vi "Module - LINX.vi"(8 "error in (no error)":errorcluster) -> (0 "error out":errorcluster)   [LabVIEW 2020]
uses:
  Control/State - LINX.ctl
  <vilib>/MakerHub/LINX/Private/Type Defs/LINX Ref.ctl
  <vilib>/MakerHub/LINX/Private/Type Defs/Platform.ctl
  <vilib>/MakerHub/LINX/Private/Type Defs/Interface.ctl
  <vilib>/MakerHub/LINX/Private/Device/Type Defs/LINX Device Config.ctl
  <vilib>/MakerHub/LINX/Private/Device/Type Defs/TCP Config.ctl
  <vilib>/MakerHub/LINX/Private/Device/Type Defs/Channels.ctl
  <vilib>/MakerHub/LINX/Private/Device/Type Defs/Wifi Config.ctl
  <vilib>/MakerHub/LINX/Private/Type Defs/WIFI Security Type.ctl
  Control/MQTT Received Data.ctl
  Control/Config File Section List.ctl
  Shared/Control/State - eFGV.ctl
  Control/MQTT Send Data.ctl
  <vilib>/numeric/Random Number (Range) U64.vi
  a823c940-d7b3-4362-9922-b3ec767b4119.vi
  <vilib>/MakerHub/LINX/Public/Peripherals/Digital/Digital Read N Chans.vi
  <vilib>/numeric/sub_Random U32.vi
  <vilib>/MakerHub/LINX/Private/Local IO/LinxDigitalRead.vi
  <vilib>/MakerHub/LINX/Public/Utilities/Check Channel.vi
  <vilib>/MakerHub/LINX/Private/Local IO/Handle Errors.vi
  <vilib>/MakerHub/LINX/Public/Utilities/Open Local.vi
  <vilib>/MakerHub/LINX/Private/Utilties/Generate Error.vi
  <userlib>/_OpenG.lib/comparison/comparison.llb/I32 Changed__ogtk.vi
  <vilib>/Comparison/Equal/Equal Functor/Equal Functor.lvclass
  <vilib>/MakerHub/LINX/LMH-LINX.lvlib
  <vilib>/MakerHub/LINX/Private/Device/Device.lvlib
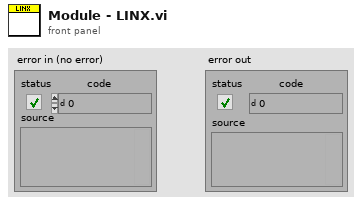
[diagram p1: front panel]
types:
  T1 = typedef "LMH-LINX.lvlib/LINX Ref.ctl" = cluster{"IO":T2, "Interface":T3, "LINX Device Config":T4}
  T2 = typedef "LMH-LINX.lvlib/Platform.ctl" = enum16{"Remote", "Local"}
  T3 = typedef "LMH-LINX.lvlib/Interface.ctl" = enum16{"Serial", "TCP"}
  T4 = typedef "LMH-LINX.lvlib/Device.lvlib/LINX Device Config.ctl" = cluster{"Interface":T3, "COM Port":refnum<visa-resource-name>, "TCP Configuration":T5, "Device Family":u8, "Device ID":u8, "Device Name":string, "TCP Ref":refnum<k5>, "Channels":T6}
  T5 = typedef "LMH-LINX.lvlib/Device.lvlib/TCP Config.ctl" = cluster{"IP Address":string, "Port":u16}
  T6 = typedef "LMH-LINX.lvlib/Channels.ctl" = cluster{"DI":u8[], "DO":u8[], "AI":u8[], "AO":u8[], "PWM":u8[], "QE":u8[], "UART":u8[], "I2C 2":u8[], "SPI":u8[], "CAN":u8[], "Servo":u8[], "AI Ref (V)":dbl, "AI Resolution (Bits)":u8, "AO Ref (V)":dbl, "AO Resolution (Bits)":u8}
  T7 = typedef "LMH-LINX.lvlib/Device.lvlib/Wifi Config.ctl" = cluster{"SSID":string, "IP Address":string, "Port":u16, "WIFI Security Type":T8, "Password":string}
  T8 = typedef "LMH-LINX.lvlib/WIFI Security Type.ctl" = enum8{"None", "WPA2 Password", "WPA2 Key", "WEP40", "WEP104"}
  T9 = typedef "MQTT Received Data.ctl" = cluster{"Receiving Module":string, "Topic":string, "Data":variant}
  T10 = cluster{"TOut":i32, "Module Name":string, "LINX Connected":bool, "User exit":bool, "Device Name":string, "LINX Resource":T1, "Wifi Configuration":T7, "Pass Counter":i32, "Reject Counter":i32, "MQTT Received Data":T9, "CK ID List":string[], "CK Defect List":string[], "CK Reject List":string[], "ID Present":bool, "Pulse per rotation":i32, "CK ID":string, "Is CK Pass?":bool, "CK ID Index":i32, "Is CK Interlock?":bool, "Extension":string}
  T11 = typedef "State - LINX.ctl" = enum16{"Init module", "Read config file", "Register for event", "Idle", "Transmit ID to Server", "Check ID in List", "Handle MQTT Event", "Create LINX Ref", "Read LINX - Digital In", "Write CK Pass", "Destroy LINX Ref", "Unregister user event", "Close module"}
  T12 = typedef "Config File Section List.ctl" = enum16{"RasPi Setting", "MQTT Server Setting", "MQTT Client Setting", "WiFi Setting", "MQTT Topics"}
  T13 = typedef "State - eFGV.ctl" = enum16{"Init", "Read", "Write", "Close"}
  T14 = typedef "MQTT Send Data.ctl" = cluster{"Sender Module":string, "Receiving Module":string, "Topic":string, "Data":variant}
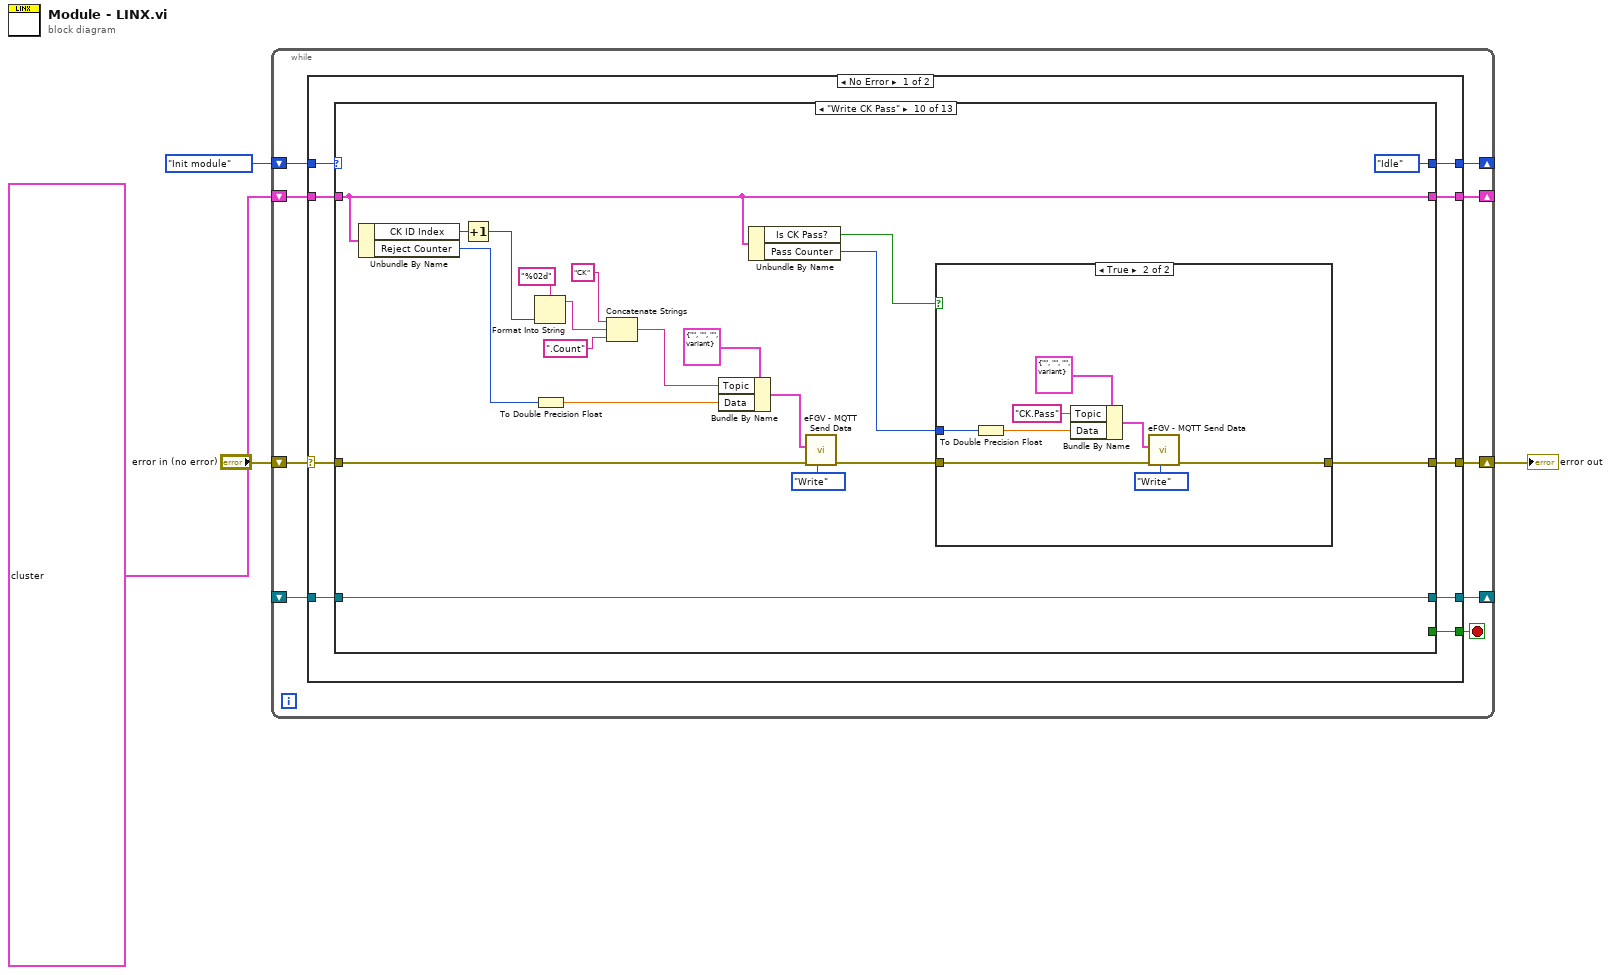
[diagram p0: block diagram]
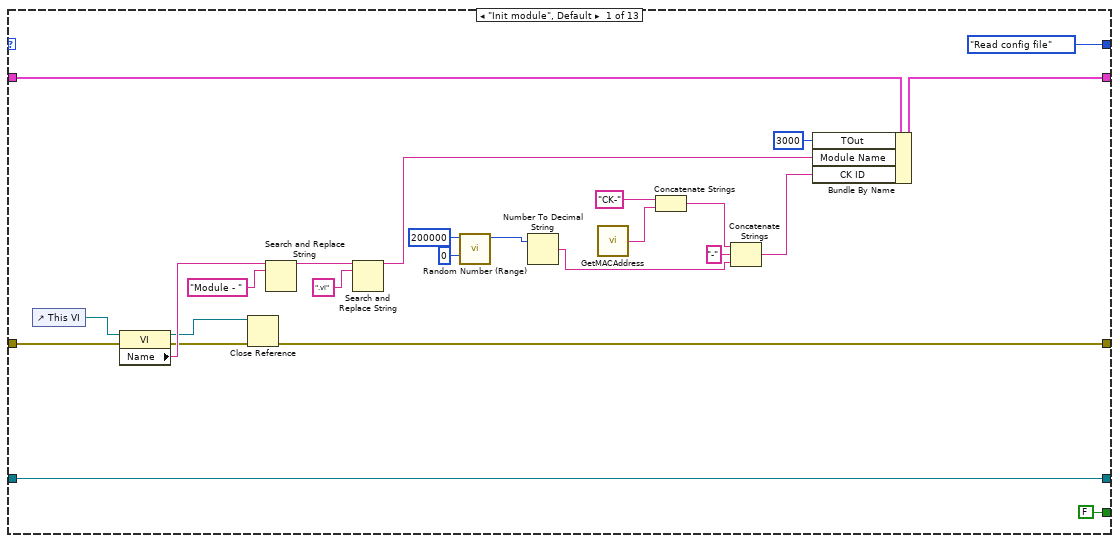
[diagram p2: hidden frame]
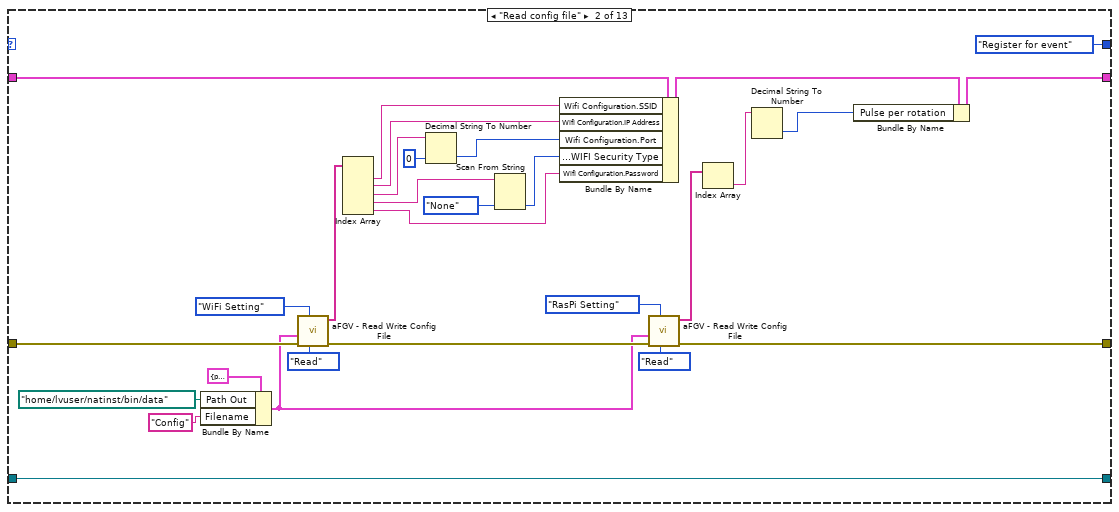
[diagram p3: hidden frame]
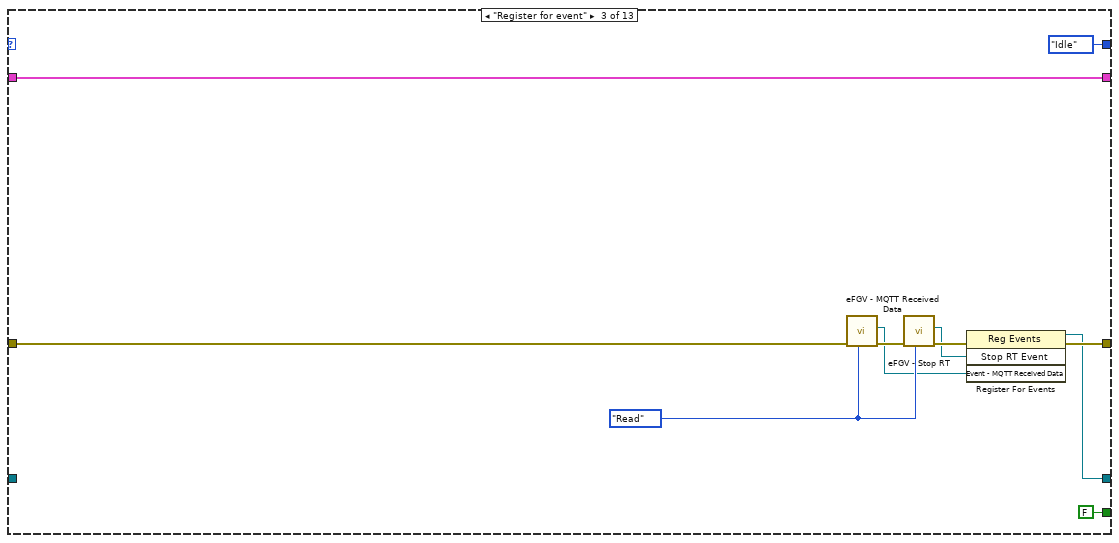
[diagram p4: hidden frame]
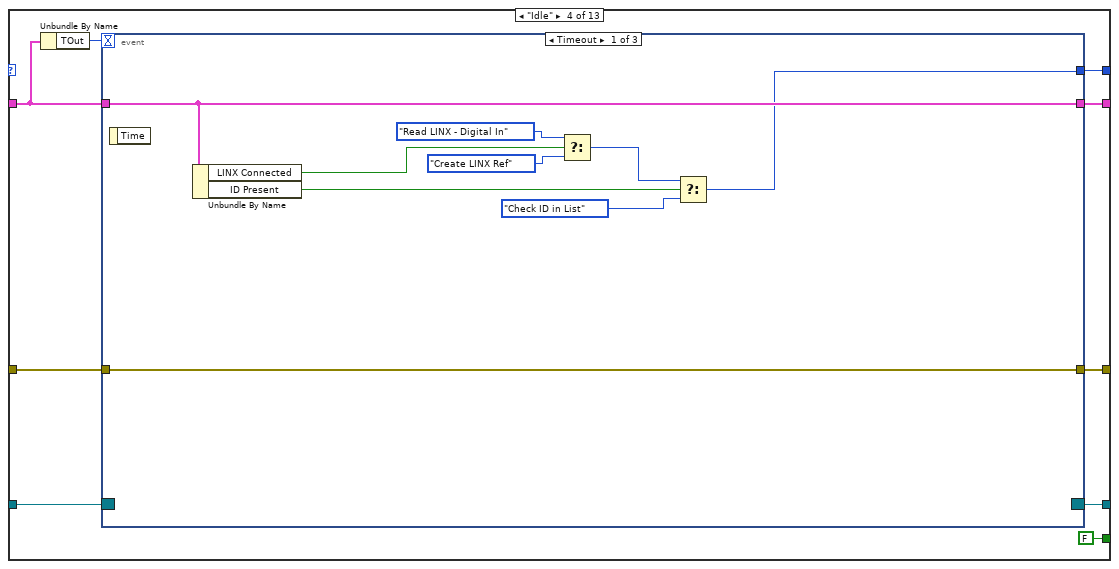
[diagram p5: hidden frame]
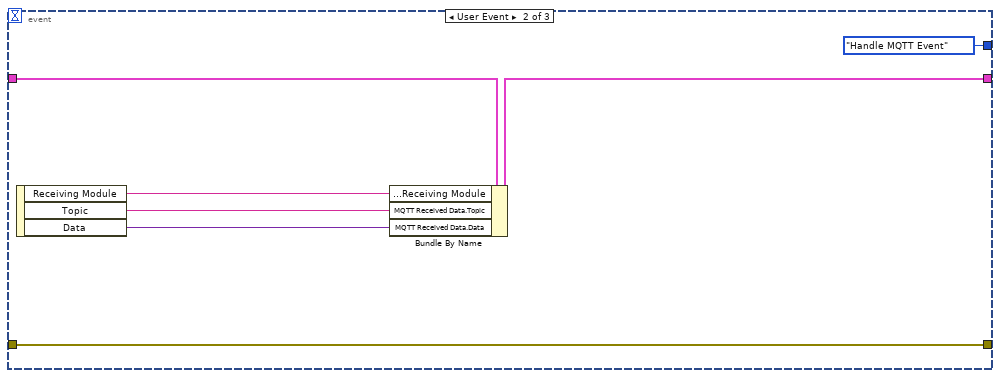
[diagram p6: hidden frame]
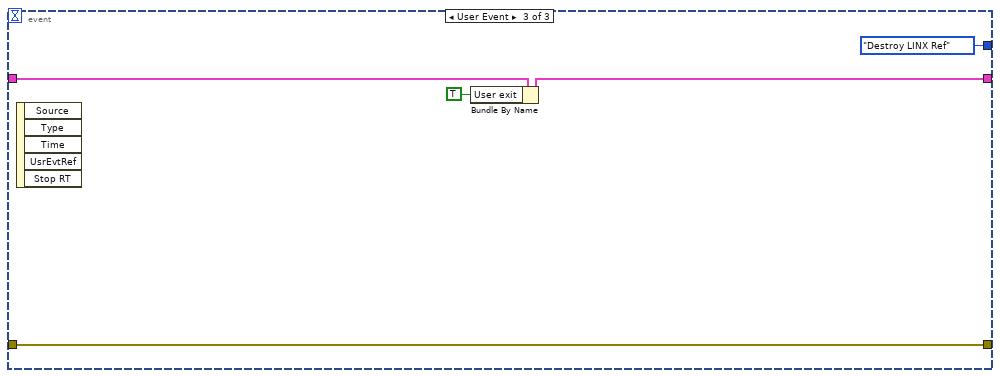
[diagram p7: hidden frame]
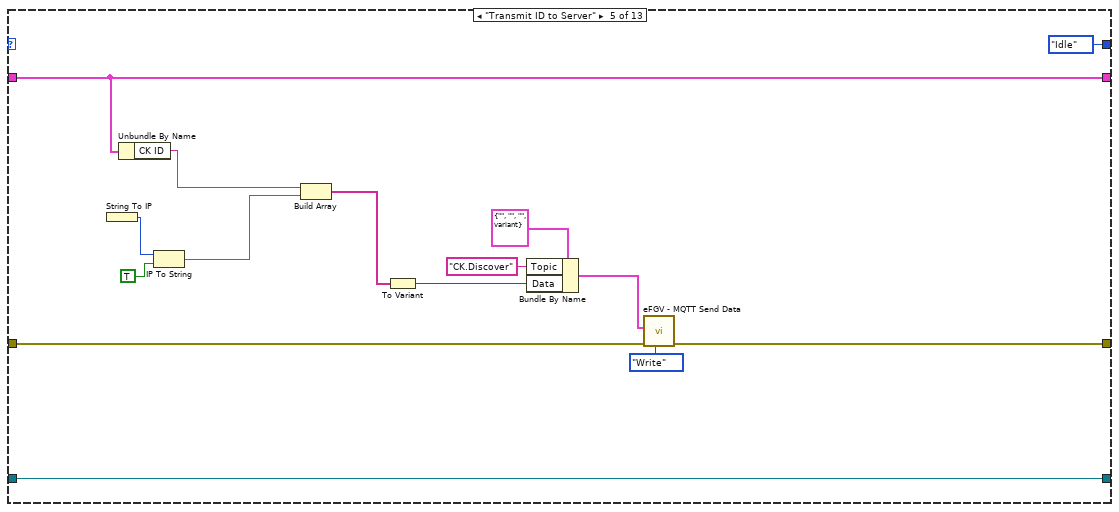
[diagram p8: hidden frame]
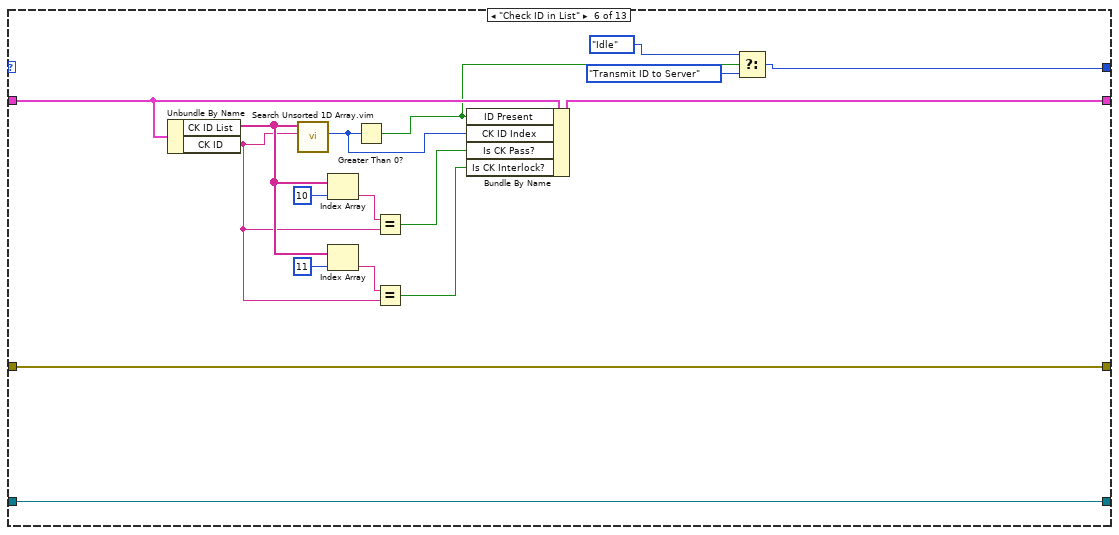
[diagram p9: hidden frame]
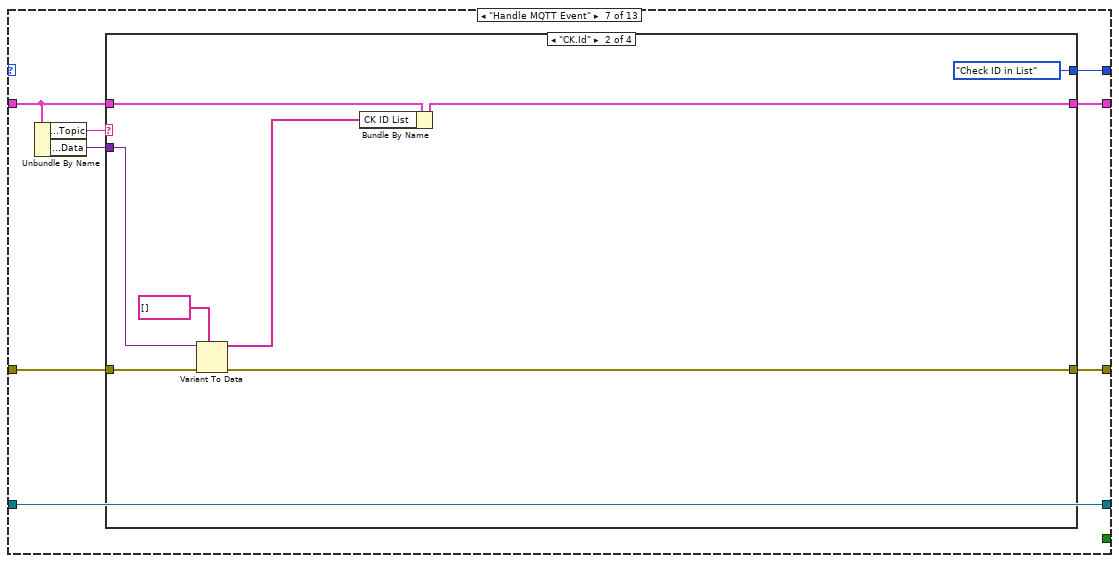
[diagram p10: hidden frame]
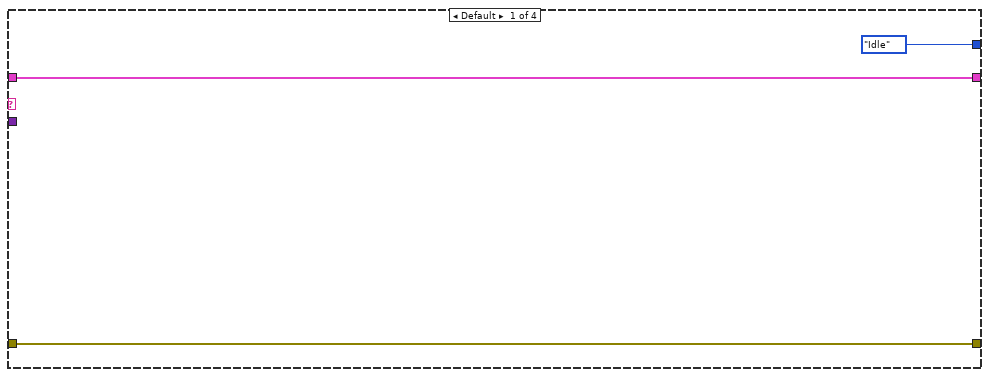
[diagram p11: hidden frame]
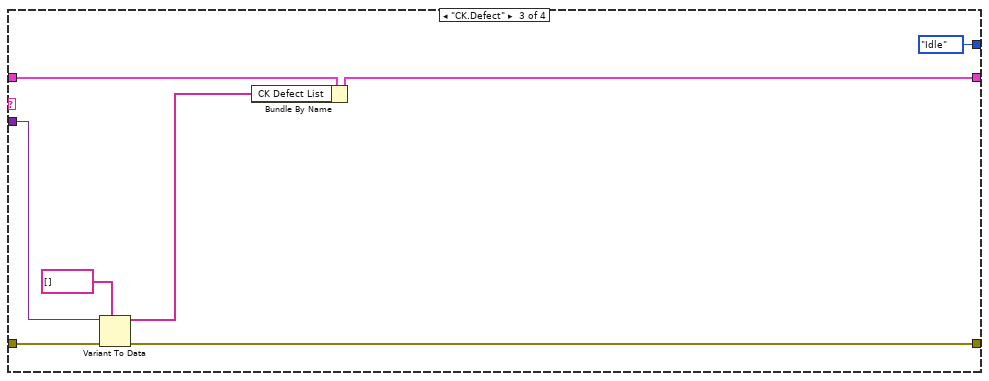
[diagram p12: hidden frame]
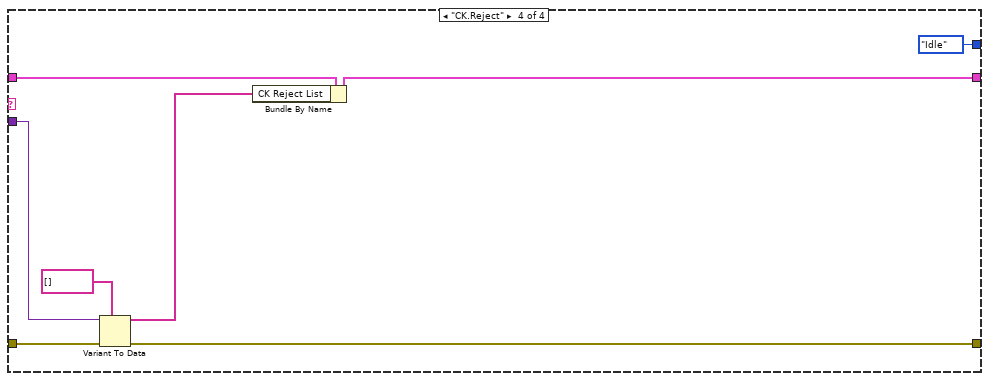
[diagram p13: hidden frame]
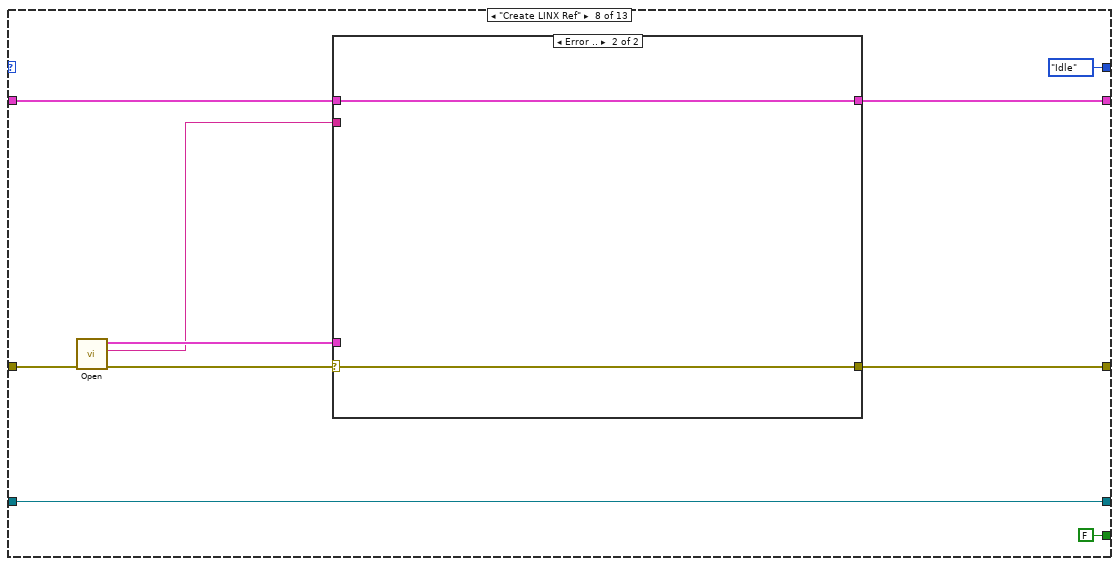
[diagram p14: hidden frame]
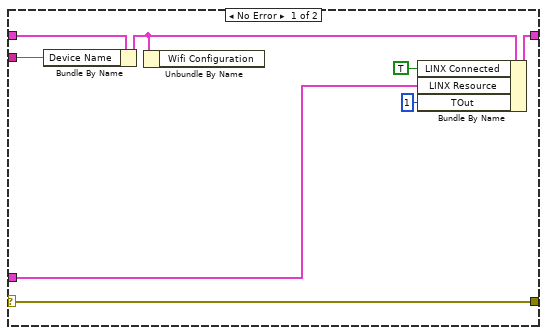
[diagram p15: hidden frame]
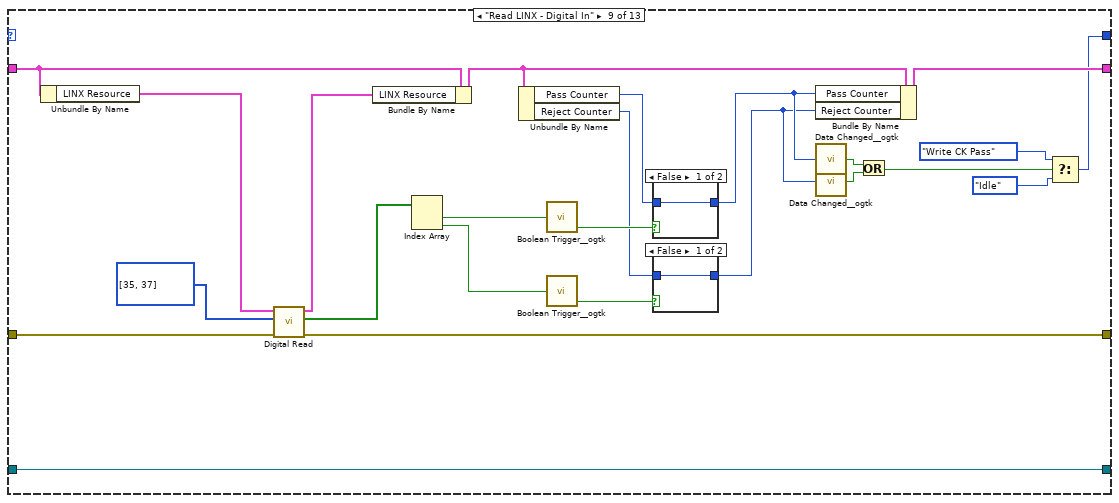
[diagram p16: hidden frame]
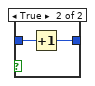
[diagram p17: hidden frame]
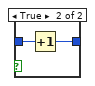
[diagram p18: hidden frame]
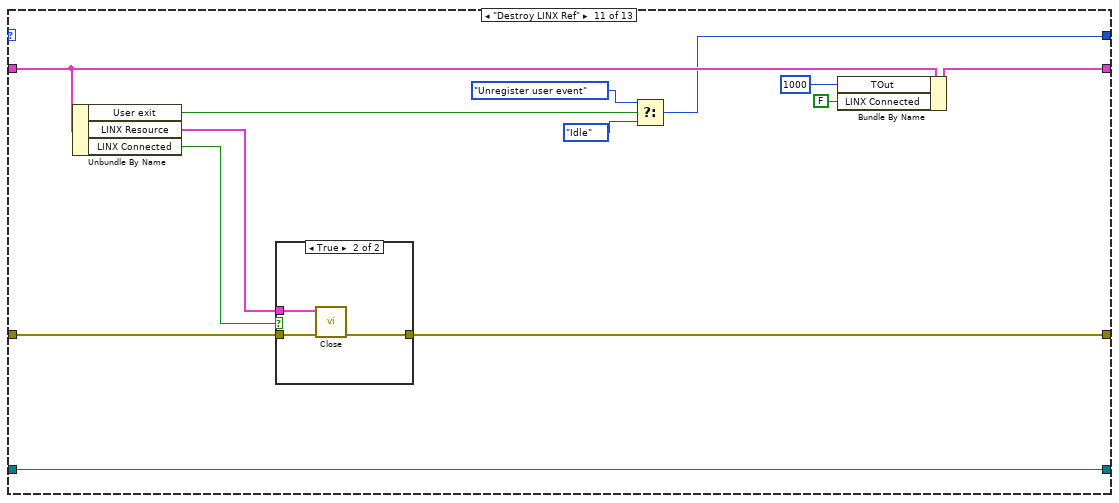
[diagram p20: hidden frame]
diagram:
  n1 = while {
    shift-right: [w9] -> w3
    shift-left: "error in (no error)" -> [w13]
    shift-right: [w5] -> _
    shift-left: State_-_LINX."Init module" -> [w11]
    shift-right: [w8] -> _
    shift-left: T10 {"TOut"=-1, "Module Name"="", "LINX Connected"=FALSE, "User exit"=FALSE, "Device Name"="", "LINX Resource"={"IO"=enum."Remote", "Interface"=enum."Serial", "LINX Device Config"={"Interface"=enum."Serial", "COM Port"="COM13", "TCP Configuration"={"IP Address"="", "Port"=0}, "Device Family"=1, "Device ID"=1, "Device Name"="myRIO-1900", "TCP Ref"=refnum, "Channels"={"DI"=[0, 1, 2, 3, 4, 5, 6, 7, 8, 9, 10, 11, 12, 13, 14, 15, 16, 17, 18, 19, 20, 21, 22, 23, 24, 25, 26, 27, 28, 29, 30, 31, 32, 33, 34, 35, 36, 37, 38, 39, 40, 41, 42, 43, 44, 45, 46], "DO"=[0, 1, 2, 3, 4, 5, 6, 7, 8, 9, 10, 11, 12, 13, 14, 15, 16, 17, 18, 19, 20, 21, 22, 23, 24, 25, 26, 27, 28, 29, 30, 31, 32, 33, 34, 35, 36, 37, 38, 39, 40, 41, 42, 43, 44, 45, 46], "AI"=[0, 1, 2, 3, 4, 5, 6, 7, 8, 9, 10, 11], "AO"=[], "PWM"=[3, 5, 6, 9, 10], "QE"=[], "UART"=[0, 1], "I2C 2"=[0], "SPI"=[0], "CAN"=[], "Servo"=[], "AI Ref (V)"=0.0, "AI Resolution (Bits)"=0, "AO Ref (V)"=0.0, "AO Resolution (Bits)"=0}}}, "Wifi Configuration"={"SSID"="VsysOEE_WiFi_BS2_5G", "IP Address"="", "Port"=0, "WIFI Security Type"=enum."WPA2 Password", "Password"="vsysoee@1"}, "Pass Counter"=0, "Reject Counter"=0, "MQTT Received Data"={"Receiving Module"="", "Topic"="", "Data"=variant}, "CK ID List"=[], "CK Defect List"=[], "CK Reject List"=[], "ID Present"=FALSE, "Pulse per rotation"=0, "CK ID"="", "Is CK Pass?"=FALSE, "CK ID Index"=0, "Is CK Interlock?"=FALSE, "Extension"=""} -> [w10]
    shift-right: [w7] -> _
    shift-left: _ -> [w6]
    stop <- w12 stop-if-true
    n2 = case shown="No Error" w13 {
      selector: w13 -> [w22 w295]
      tunnel: [w21 FALSE] -> w12
      tunnel: w11 -> [w20 _]
      tunnel: w10 -> [w19 w293]
      tunnel: [w18 w294] -> w9
      tunnel: [w17 w293] -> w8
      tunnel: [w16 w296] -> w7
      tunnel: w6 -> [w15 w296]
      tunnel: [w14 State_-_LINX."Destroy LINX Ref" ("f")] -> w5
      frame No Error {
        n3 = case shown="\"Write CK Pass\"" w20 {
          tunnel: w22 -> [w37 w68 w79 w94 w130 w149 w154 w191 w226 w251 w274 w285 w291]
          tunnel: [FALSE _ FALSE FALSE _ _ _ FALSE _ _ _ FALSE TRUE] -> w21
          tunnel: w19 -> [w46 w76 w84 w91 w126 w147 w153 w194 w227 w240 w275 w286 w290]
          tunnel: [w36 w53 w86 w93 w129 w149 w152 w190 w221 w238 w273 w284 w291] -> w18
          tunnel: [w35 w52 w84 w90 w126 w144 w151 w187 w214 w240 w267 w286 w290] -> w17
          tunnel: [w45 w75 w85 w95 w132 w148 w157 w193 w228 w254 w276 w283 w289] -> w16
          tunnel: w15 -> [w45 w75 _ w96 w132 w148 w157 w193 w228 w254 w276 w283 w289]
          tunnel: [State_-_LINX."Read config file" State_-_LINX."Register for event" ("f") State_-_LINX."Idle" w88 State_-_LINX."Idle" ("f") w133 w150 State_-_LINX."Idle" ("f") w205 State_-_LINX."Idle" ("f") w268 State_-_LINX."Close module" ("f") State_-_LINX."Close module" ("f")] -> w14
          frame "Init module", Default {
            n4 = control-ref of="This VI"() -> (w44:refnum<vi>)
            n5 = property class="VI"(reference=w44, error in=w37) -> (reference out=w38:refnum<vi>, error out=w39:errorcluster, "Name"=w43:string)
            n6 = Close Reference(reference=w38, error in (no error)=w39) -> (error out=w36:errorcluster)
            n7 = Search and Replace String(input string=w43, search string="Module - ") -> (result string=w40:string)  [unwired: 6 in, 3 out]
            n8 = Search and Replace String(input string=w40, search string=".vi") -> (result string=w34:string)  [unwired: 6 in, 3 out]
            n9 = call-poly <vilib>:"Random Number (Range).vi"("lower bound (0)"=u64 0, "upper bound (100)"=u64 200000) -> ("number"=w29:u64)  [unwired: 9 in]
            n10 = Number To Decimal String(number=w29) -> (decimal integer string=w24:string)  [unwired: 1 in]
            n11 = call "GetMACAddress.vi"() -> ("MAC Address"=w27:string)  [unwired: 1 in]
            n12 = Concatenate Strings("CK-" ("string"), w27) -> (w26:string)
            n13 = Concatenate Strings(w26, "-" ("string"), w24) -> (w23:string)
            n14 = Bundle By Name(cluster=w46, "TOut"=3000, "Module Name"=w34, "CK ID"=w23) -> (w35:T10)
          }
          frame "Read config file" {
            n15 = Bundle By Name(cluster=cluster{"Path Out":path, "Filename":string} {"Path Out"=path "", "Filename"=""} ("Path File"), "Path Out"=path "/home/lvuser/natinst/bin/data", "Filename"="Config") -> (w48:cluster{"Path Out":path, "Filename":string})
            n16 = call "aFGV - Read Write Config File.vi"("State"=enum16{"Read", "Write", "Delete"}."Read", "Section"=Config_File_Section_List."WiFi Setting", "Error In"=w68, "Path File"=w48) -> ("Error Out"=w54:errorcluster, "Data out"=w67:string[])  [unwired: 5 in, 1 out]
            n17 = Index Array(array=w67) -> (element #1=w65:string, element #2=w64:string, element #3=w63:string, element #4=w61:string, element #5=w57:string)  [unwired: 5 in]
            n18 = Decimal String To Number(string=w63, default (0L)=u16 0 ("Wifi Configuration.Port")) -> (number=w59:u16)  [unwired: 1 in, 1 out]
            n19 = Scan From String(input string=w61, default 1=WIFI_Security_Type."None" ("Wifi Configuration.WIFI Security Type")) -> (output 1=w58:T8)  [unwired: 3 in, 3 out]
            n20 = Bundle By Name(cluster=w76, "Wifi Configuration.SSID"=w65, "Wifi Configuration.IP Address"=w64, "Wifi Configuration.Port"=w59, "Wifi Configuration.WIFI Security Type"=w58, "Wifi Configuration.Password"=w57) -> (w66:T10)
            n21 = call "aFGV - Read Write Config File.vi"("State"=enum16{"Read", "Write", "Delete"}."Read", "Section"=Config_File_Section_List."RasPi Setting", "Error In"=w54, "Path File"=w48) -> ("Error Out"=w53:errorcluster, "Data out"=w51:string[])  [unwired: 5 in, 1 out]
            n22 = Index Array(array=w51) -> (element=w49:string)  [unwired: 1 in]
            n23 = Decimal String To Number(string=w49) -> (number=w50:i32)  [unwired: 2 in, 1 out]
            n24 = Bundle By Name(cluster=w66, "Pulse per rotation"=w50) -> (w52:T10)
          }
          frame "Register for event" {
            w78 = State_-_eFGV."Read" ("State")
            n25 = call "eFGV - MQTT Received Data.vi"("State"=w78, "error in (no error)"=w79) -> ("error out"=w80:errorcluster, "Event - MQTT Received Data"=w77:refnum<user-event>)  [unwired: 8 in]
            n26 = call "eFGV - Stop RT.vi"("State"=w78, "error in (no error)"=w80) -> ("error out"=w82:errorcluster, "Stop RT Event"=w81:refnum<user-event>)  [unwired: 8 in]
            n27 = register-events(error in=w82, w81, w77) -> (reference out=w85:refnum<event-registration>, error out=w86:errorcluster)  [unwired: 1 in]
          }
          frame "Idle" {
            n28 = Unbundle By Name(w91) -> ("TOut"=w92:i32)
            n29 = event shown="[0] Timeout" {
              selector: w96 -> [_ _ _]
              dyn-events: [_ _ _] -> w95
              timeout: w92 -> [_ _ _]
              tunnel: w94 -> [w105 w112 w115]
              tunnel: [w105 w112 w115] -> w93
              tunnel: w91 -> [w104 w110 w116]
              tunnel: [w104 w109 w114] -> w90
              tunnel: [w103 State_-_LINX."Handle MQTT Event" ("f") State_-_LINX."Destroy LINX Ref" ("f")] -> w88
              event Timeout {
                n30 = event-data() -> ()  [unwired: 1 in, 1 out]
                n31 = Unbundle By Name(w104) -> ("LINX Connected"=w100:bool, "ID Present"=w102:bool)
                n32 = Select(t=State_-_LINX."Read LINX - Digital In", s=w100, f=State_-_LINX."Create LINX Ref") -> (s? t:f=w99:T11)
                n33 = Select(t=w99, s=w102, f=State_-_LINX."Check ID in List") -> (s? t:f=w103:T11)
              }
              event User Event {
                n34 = event-data() -> ("Receiving Module"=w108:string, "Topic"=w107:string, "Data"=w106:variant)  [unwired: 1 in]
                n35 = Bundle By Name(cluster=w110, "MQTT Received Data.Receiving Module"=w108, "MQTT Received Data.Topic"=w107, "MQTT Received Data.Data"=w106) -> (w109:T10)
              }
              event User Event {
                n36 = event-data() -> ()  [unwired: 1 in, 5 out]
                n37 = Bundle By Name(cluster=w116, "User exit"=TRUE) -> (w114:T10)
              }
            }
          }
          frame "Transmit ID to Server" {
            n38 = String To IP() -> (0:w123:u32)  [unwired: 1 in]
            n39 = Unbundle By Name(w126) -> ("CK ID"=w118:string)
            n40 = IP To String(1:TRUE ("dot notation? (F)"), 2:w123) -> (0:w121:string)
            n41 = Build Array(w118, w121) -> (w120:string[])
            n42 = To Variant(anything=w120) -> (Variant=w119:variant)
            n43 = Bundle By Name(cluster=T14 {"Sender Module"="", "Receiving Module"="", "Topic"="", "Data"=variant} ("MQTT Send Data"), "Topic"="CK.Discover", "Data"=w119) -> (w127:T14)
            n44 = call "eFGV - MQTT Send Data.vi"("State"=State_-_eFGV."Write", "error in (no error)"=w130, "MQTT Send Data"=w127) -> ("error out"=w129:errorcluster)  [unwired: 7 in, 1 out]
          }
          frame "Check ID in List" {
            n45 = Unbundle By Name(w147) -> ("CK ID List"=w139:string[], "CK ID"=w138:string)
            n46 = call "Search Unsorted 1D Array.vim"("element"=w138, "unsorted 1D array"=w139) -> ("index of element"=w143:i32)  [unwired: 9 in]
            n47 = Index Array(array=w139, index=10) -> (element=w145:string)
            n48 = Index Array(array=w139, index=11) -> (element=w141:string)
            n49 = Greater Than 0?(x=w143) -> (x > 0?=w136:bool)
            n50 = Equal?(x=w145, y=w138) -> (x = y?=w142:bool)
            n51 = Equal?(x=w141, y=w138) -> (x = y?=w137:bool)
            n52 = Bundle By Name(cluster=w147, "ID Present"=w136, "CK ID Index"=w143, "Is CK Pass?"=w142, "Is CK Interlock?"=w137) -> (w144:T10)
            n53 = Select(t=State_-_LINX."Idle" ("f"), s=w136, f=State_-_LINX."Transmit ID to Server") -> (s? t:f=w133:T11)
          }
          frame "Handle MQTT Event" {
            n54 = Unbundle By Name(w153) -> ("MQTT Received Data.Topic"=w156:string, "MQTT Received Data.Data"=w155:variant)
            n55 = case shown="\"CK.Id\"" w156 {
              tunnel: w155 -> [_ w165 w173 w181]
              tunnel: w154 -> [w160 w167 w175 w183]
              tunnel: w153 -> [w159 w168 w176 w184]
              tunnel: [w160 w166 w174 w182] -> w152
              tunnel: [w159 w163 w171 w179] -> w151
              tunnel: [State_-_LINX."Idle" State_-_LINX."Check ID in List" State_-_LINX."Idle" State_-_LINX."Idle"] -> w150
              frame Default {
              }
              frame "CK.Id" {
                n56 = Variant To Data(error in=w167, type=string[] [], Variant=w165) -> (data=w162:string[], error out=w166:errorcluster)
                n57 = Bundle By Name(cluster=w168, "CK ID List"=w162) -> (w163:T10)
              }
              frame "CK.Defect" {
                n58 = Variant To Data(error in=w175, type=string[] [], Variant=w173) -> (data=w170:string[], error out=w174:errorcluster)
                n59 = Bundle By Name(cluster=w176, "CK Defect List"=w170) -> (w171:T10)
              }
              frame "CK.Reject" {
                n60 = Variant To Data(error in=w183, type=string[] [], Variant=w181) -> (data=w178:string[], error out=w182:errorcluster)
                n61 = Bundle By Name(cluster=w184, "CK Reject List"=w178) -> (w179:T10)
              }
            }
          }
          frame "Create LINX Ref" {
            n62 = call-poly <vilib>:"Open.vi"("Error In"=w191) -> ("Error Out"=w186:errorcluster, "Device Name"=w188:string, "LINX Resource"=w189:T1)  [unwired: 8 in]
            n63 = case shown="Error .." w186 {
              selector: w186 -> [w197 w203]
              tunnel: w194 -> [w202 w204]
              tunnel: [w197 w203] -> w190
              tunnel: w189 -> [w201 _]
              tunnel: w188 -> [w200 _]
              tunnel: [w198 w204] -> w187
              frame No Error {
                n64 = Bundle By Name(cluster=w202, "Device Name"=w200) -> (w199:T10)
                n65 = Unbundle By Name(w199) -> ()  [unwired: 1 out]
                n66 = Bundle By Name(cluster=w199, "LINX Connected"=TRUE, "LINX Resource"=w201, "TOut"=1) -> (w198:T10)
              }
              frame Error {
              }
            }
          }
          frame "Read LINX - Digital In" {
            n67 = Unbundle By Name(w227) -> ("LINX Resource"=w225:T1)
            n68 = call-poly <vilib>:"Digital Read.vi"("Error In"=w226, "DI Channels"=u8[] [35, 37], "LINX Resource"=w225) -> ("Error Out"=w221:errorcluster, "Values"=w223:bool[], "LINX Resource"=w222:T1)  [unwired: 6 in]
            n69 = Bundle By Name(cluster=w227, "LINX Resource"=w222) -> (w213:T10)
            n70 = Index Array(array=w223) -> (element #1=w220:bool, element #2=w219:bool)  [unwired: 2 in]
            n71 = Unbundle By Name(w213) -> ("Pass Counter"=w215:i32, "Reject Counter"=w216:i32)
            n72 = call <userlib>:"Boolean Trigger__ogtk.vi"("Boolean Input"=w220) -> ("Falling Edge"=w218:bool)  [unwired: 1 in, 1 out]
            n73 = call <userlib>:"Boolean Trigger__ogtk.vi"("Boolean Input"=w219) -> ("Falling Edge"=w217:bool)  [unwired: 1 in, 1 out]
            n74 = case shown="False" w218 {
              tunnel: w215 -> [w232 w234]
              tunnel: [w232 w233] -> w212
              frame False {
              }
              frame True {
                n75 = Increment(x=w234) -> (x+1=w233:i32)
              }
            }
            n76 = case shown="False" w217 {
              tunnel: w216 -> [w229 w231]
              tunnel: [w229 w230] -> w211
              frame False {
              }
              frame True {
                n77 = Increment(x=w231) -> (x+1=w230:i32)
              }
            }
            n78 = Bundle By Name(cluster=w213, "Pass Counter"=w212, "Reject Counter"=w211) -> (w214:T10)
            n79 = call-poly <userlib>:"Data Changed__ogtk.vi"("I32"=w212) -> ("Changed"=w210:bool)
            n80 = call-poly <userlib>:"Data Changed__ogtk.vi"("I32"=w211) -> ("Changed"=w209:bool)
            n81 = Or(x=w210, y=w209) -> (x .or. y?=w208:bool)
            n82 = Select(t=State_-_LINX."Write CK Pass" ("f"), s=w208, f=State_-_LINX."Idle") -> (s? t:f=w205:T11)
          }
          frame "Write CK Pass" {
            n83 = Unbundle By Name(w240) -> ("CK ID Index"=w249:i32, "Reject Counter"=w241:i32)
            n84 = Increment(x=w249) -> (x+1=w247:i32)
            n85 = Format Into String(format string="%02d", w247) -> (resulting string=w244:string)  [unwired: 2 in, 1 out]
            n86 = To Double Precision Float(number=w241) -> (double precision float=w235:dbl)
            n87 = Concatenate Strings("CK" ("string"), w244, ".Count" ("string")) -> (w242:string)
            n88 = Bundle By Name(cluster=T14 {"Sender Module"="", "Receiving Module"="", "Topic"="", "Data"=variant} ("MQTT Send Data"), "Topic"=w242, "Data"=w235) -> (w253:T14)
            n89 = Unbundle By Name(w240) -> ("Is CK Pass?"=w237:bool, "Pass Counter"=w236:i32)
            n90 = call "eFGV - MQTT Send Data.vi"("State"=State_-_eFGV."Write", "error in (no error)"=w251, "MQTT Send Data"=w253) -> ("error out"=w239:errorcluster)  [unwired: 7 in, 1 out]
            n91 = case shown="True" w237 {
              tunnel: w239 -> [w255 w260]
              tunnel: [w255 w258] -> w238
              tunnel: w236 -> [_ w257]
              frame False {
              }
              frame True {
                n92 = To Double Precision Float(number=w257) -> (double precision float=w256:dbl)
                n93 = Bundle By Name(cluster=T14 {"Sender Module"="", "Receiving Module"="", "Topic"="", "Data"=variant} ("MQTT Send Data"), "Topic"="CK.Pass", "Data"=w256) -> (w259:T14)
                n94 = call "eFGV - MQTT Send Data.vi"("State"=State_-_eFGV."Write", "error in (no error)"=w260, "MQTT Send Data"=w259) -> ("error out"=w258:errorcluster)  [unwired: 7 in, 1 out]
              }
            }
          }
          frame "Destroy LINX Ref" {
            n95 = Unbundle By Name(w275) -> ("User exit"=w271:bool, "LINX Resource"=w272:T1, "LINX Connected"=w264:bool)
            n96 = case shown="True" w264 {
              tunnel: w274 -> [w277 w280]
              tunnel: [w277 w279] -> w273
              tunnel: w272 -> [_ w278]
              frame False {
              }
              frame True {
                n97 = call <vilib>:"Close.vi"("Error In"=w280, "LINX Resource"=w278) -> ("Error Out"=w279:errorcluster)  [unwired: 9 in]
              }
            }
            n98 = Select(t=State_-_LINX."Unregister user event" ("f"), s=w271, f=State_-_LINX."Idle") -> (s? t:f=w268:T11)
            n99 = Bundle By Name(cluster=w275, "TOut"=1000, "LINX Connected"=FALSE) -> (w267:T10)
          }
          frame "Unregister user event" {
            n100 = Unregister For Events(event registration refnum=w283, error in=w285) -> (error out=w284:errorcluster)
          }
          frame "Close module" {
          }
        }
      }
      frame Error {
        n101 = call <vilib>:"Clear Errors.vi"("error in (no error)"=w295) -> ("error out"=w294:errorcluster)  [unwired: 5 in, 1 out]
      }
    }
  }
  "error out" <- w3
